vi "Encode Secret.vi"(10 "Secret":string) -> (2 "Encoded Secret":string)   [LabVIEW 2013, in "Connection.WS_GOSPL.lvlib" / "Connection.WS.lvclass"]
uses:
  Connection.WS.lvclass
  <vilib>/LabVIEW Open Source Project/Cryptographic Functions/SHA-1/SHA-1.lvclass
  <vilib>/LabVIEW Open Source Project/OpenSerializer.Base64/Base64_CharSet.vi
  <vilib>/LabVIEW Open Source Project/OpenSerializer.Base64/Serializer.Base64.lvclass
  <vilib>/LabVIEW Open Source Project/Cryptographic Functions/SHA-1/SHA-1.lvlib
panel:
  # "EXAMPLE\n\nSecret: \ndGhlIHNhbXBsZSBub25jZQ==\n\nEncoded Secret: \ns3pPLMBiTxaQ9kYGzzhZRbK+xOo="
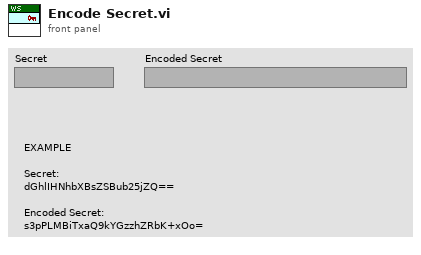
[diagram p1: front panel]
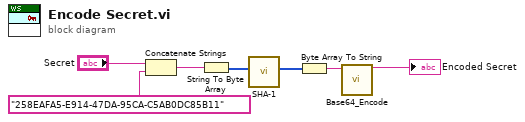
[diagram p0: block diagram]
diagram:
  n1 = Concatenate Strings("Secret", "258EAFA5-E914-47DA-95CA-C5AB0DC85B11") -> (w1:string)
  n2 = String To Byte Array(string=w1) -> (unsigned byte array=w4:u8[])
  n3 = call <vilib>:"SHA-1.vi"("data"=w4) -> ("SHA-1 hash"=w3:u8[])  [unwired: 10 in]
  n4 = Byte Array To String(unsigned byte array=w3) -> (string=w2:string)
  n5 = call <vilib>:"Base64_Encode.vi"("String"=w2) -> ("Encoded String"=→"Encoded Secret":string)  [unwired: 9 in, 1 out]
